vi "Name.vi"(11 "List Data Type in":refnum<class "List Data Type.lvclass">) -> (2 "String":string="Generic", 3 "List Data Type (dup)":refnum<class "List Data Type.lvclass">)   [LabVIEW 2018, in "List Data Type.lvclass"]
uses:
  List Data Type.lvclass
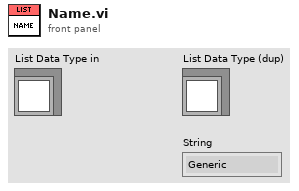
[diagram p1: front panel]
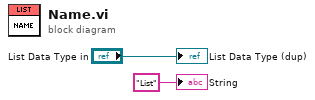
[diagram p0: block diagram]
diagram:
  "List Data Type (dup)" <- "List Data Type in"
  "String" <- "List" ("String")
